vi "subLoad_ConstrutLabVIEWItem.vi"(11 "Caller path":path) -> (3 "Params":T1[](array[typedef]))   [LabVIEW 2020, in "Tests.LabVIEWItem.lvlib"]
uses:
  Tests.LabVIEWItem.lvlib
  Validation/Params_ConstructLabVIEWItem.ctl
  Validation/Input_BaseConstruction.ctl
  Validation/Validate_BaseConstruction.ctl
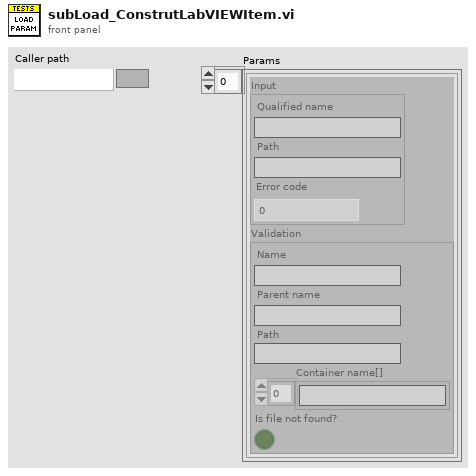
[diagram p1: front panel]
types:
  T1 = typedef "Tests.LabVIEWItem.lvlib/Params_ConstructLabVIEWItem.ctl" = cluster{"Input":T2, "Validation":T3}
  T2 = typedef "Tests.LabVIEWItem.lvlib/Input_BaseConstruction.ctl" = cluster{"Qualified name":string, "Path":string, "Error code":i32}
  T3 = typedef "Tests.LabVIEWItem.lvlib/Validate_BaseConstruction.ctl" = cluster{"Name":string, "Parent name":string, "Path":string, "Container name[]":string[], "Is file not found?":bool}
  T4 = enum16{"open", "replace", "create", "open or create", "replace or create", "replace or create with confirmation"}
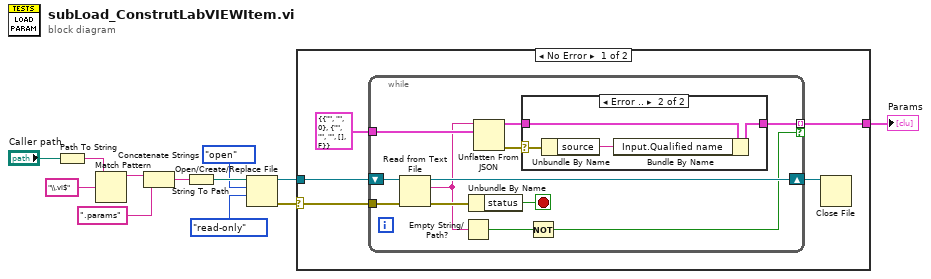
[diagram p0: block diagram]
diagram:
  n1 = Path To String(path="Caller path") -> (string=w8:string)
  n2 = Match Pattern(string=w8, regular expression="\\.vi$") -> (before substring=w11:string)  [unwired: 1 in, 3 out]
  n3 = Concatenate Strings(w11, ".params" ("string")) -> (w7:string)
  n4 = String To Path(string=w7) -> (path=w6:path)
  n5 = Open/Create/Replace File(file path (use dialog)=w6, operation (0:open)=T4."open", access (0:read/write)=enum16{"read/write", "read-only", "write-only"}."read-only") -> (refnum out=w3:refnum<file>, error out=w2:errorcluster)  [unwired: 3 in, 1 out]
  n6 = case shown="No Error" w2 {
    selector: w2 -> [w16 _]
    tunnel: w3 -> [w17 _]
    tunnel: [w15 _] -> w1
    frame No Error {
      n7 = while {
        tunnel: T1 {"Input"={"Qualified name"="", "Path"="", "Error code"=0}, "Validation"={"Name"="", "Parent name"="", "Path"="", "Container name[]"=[], "Is file not found?"=FALSE}} -> [w29]
        tunnel: w16 -> [w27]
        shift-right: [w26] -> w13
        shift-left: w17 -> [w28]
        tunnel: [w19] -> w15 mode=indexing if=w25
        stop <- w22 stop-if-true
        n8 = Read from Text File(file (use dialog)=w28, error in=w27) -> (refnum out=w26:refnum<file>, text=w23:string, error out=w24:errorcluster)  [unwired: 2 in, 1 out]
        n9 = Empty String/Path?(string/path=w23) -> (empty?=w21:bool)
        n10 = Unbundle By Name(w24) -> ("status"=w22:bool)
        n11 = Unflatten From JSON(JSON string=w23, type and defaults=w29) -> (value=w18:T1, error out=w20:errorcluster)  [unwired: 5 in]
        n12 = case shown="Error .." w20 {
          selector: w20 -> [_ w34]
          tunnel: [w30 w32] -> w19
          tunnel: w18 -> [w30 w33]
          frame No Error {
          }
          frame Error {
            n13 = Unbundle By Name(w34) -> ("source"=w31:string)
            n14 = Bundle By Name(cluster=w33, "Input.Qualified name"=w31) -> (w32:T1)
          }
        }
        n15 = Not(x=w21) -> (.not. x?=w25:bool)
      }
      n16 = Close File(refnum=w13) -> ()  [unwired: 1 in, 2 out]
    }
    frame Error {
    }
  }
  "Params" <- w1
